vi "File Write with Filename.vi"(0 "Path":path, 5 "text":string, 11 "error in":errorcluster) -> (4 "path":path, 15 "error out":errorcluster)   [LabVIEW 2012]
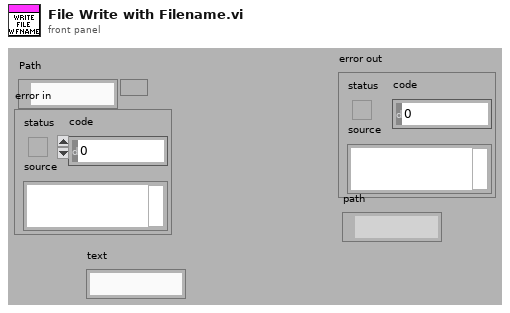
[diagram p1: front panel]
types:
  T1 = enum16{"open", "replace", "create", "open or create", "replace or create", "replace or create with confirmation"}
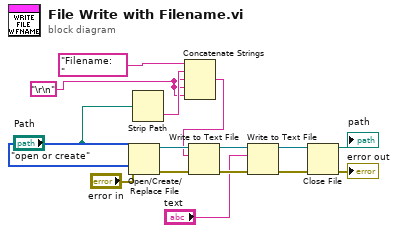
[diagram p0: block diagram]
diagram:
  w1 = "\r\n"
  n1 = Open/Create/Replace File(file path (use dialog)="Path", error in="error in", operation (0:open)=T1."open or create") -> (refnum out=w12:refnum<file>, error out=w15:errorcluster)  [unwired: 3 in, 1 out]
  n2 = Strip Path(path="Path") -> (name=w4:string)  [unwired: 1 out]
  n3 = Concatenate Strings("Filename:     " ("string"), w4, w1, w1, w1) -> (w3:string)
  n4 = Write to Text File(file (use dialog)=w12, text=w3, error in=w15) -> (refnum out=w11:refnum<file>, error out=w16:errorcluster)  [unwired: 1 in, 1 out]
  n5 = Write to Text File(file (use dialog)=w11, text="text", error in=w16) -> (refnum out=w13:refnum<file>, error out=w14:errorcluster)  [unwired: 1 in, 1 out]
  n6 = Close File(refnum=w13, error in=w14) -> (path=→"path":path, error out=→"error out":errorcluster)
